vi "INFOOFMOTOR.vi"(9 "input cluster":T1, 10 "reference in":refnum<vi>, 11 "Array in":refnum<vi>) -> (3 "Mirror Info":string[](array[string]))   [LabVIEW 2013]
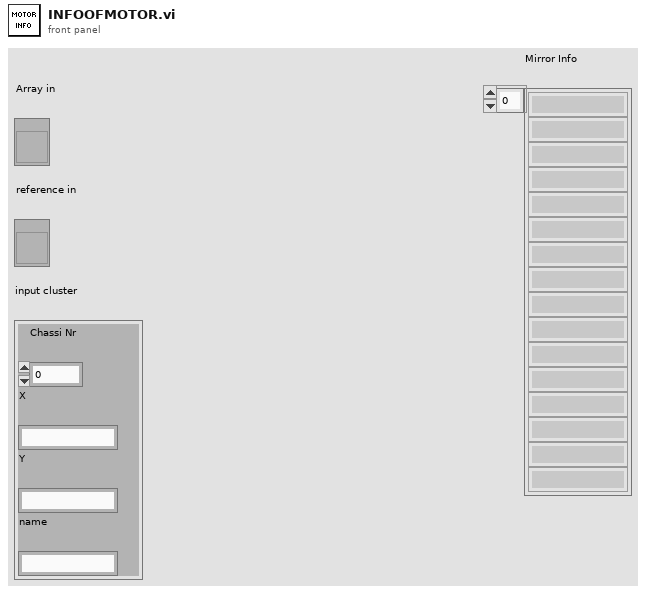
[diagram p1: front panel]
types:
  T1 = cluster{"Chassi Nr":i32, "X":string, "Y":string, "name":string}
  T2 = typedef "TRAServer.lvclass/StatusTRA_TypDef.ctl" = enum16{"NOT REFERENCED", "CONFIGURATION", "HOMING", "MOVING", "READY", "DISABLE", "JOGGING"}
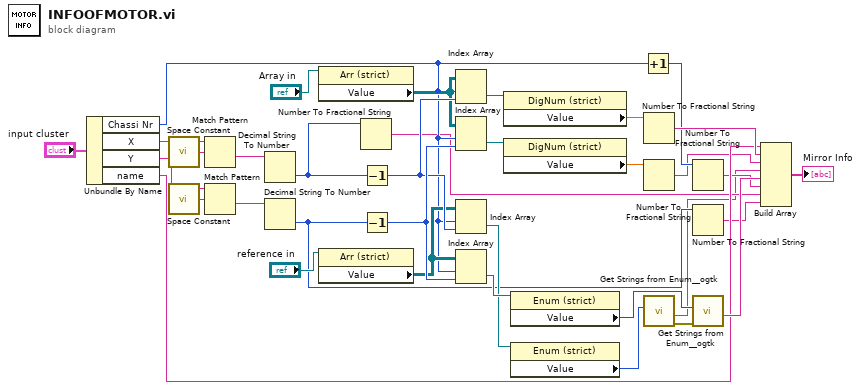
[diagram p0: block diagram]
diagram:
  n1 = Unbundle By Name("input cluster") -> ("Chassi Nr"=w9:i32, "X"=w16:string, "Y"=w20:string, "name"=w33:string)
  n2 = call <vilib>:"Space Constant.vi"() -> ("String"=w15:string)
  n3 = call <vilib>:"Space Constant.vi"() -> ("String"=w18:string)
  n4 = Match Pattern(string=w16, regular expression=w15) -> (after substring=w14:string)  [unwired: 1 in, 3 out]
  n5 = Match Pattern(string=w20, regular expression=w18) -> (after substring=w19:string)  [unwired: 1 in, 3 out]
  n6 = Decimal String To Number(string=w14) -> (number=w5:i32)  [unwired: 2 in, 1 out]
  n7 = Decimal String To Number(string=w19) -> (number=w6:i32)  [unwired: 2 in, 1 out]
  n8 = property class="Arr (strict)"(reference="Array in") -> ("Value"=w17:refnum<vi>[][])  [unwired: 1 in, 2 out]
  n9 = property class="Arr (strict)"(reference="reference in") -> ("Value"=w22:refnum<vi>[][])  [unwired: 1 in, 2 out]
  n10 = Number To Fractional String(number=w5) -> (F-format string=w3:string)  [unwired: 3 in]
  n11 = Decrement(x=w5) -> (x-1=w23:i32)
  n12 = Decrement(x=w6) -> (x-1=w24:i32)
  n13 = Index Array(array=w17, index (row)=w9, index (col)=w23) -> (element=w13:refnum<vi>)
  n14 = Index Array(array=w17, index (row)=w9, index (col)=w24) -> (element=w21:refnum<vi>)
  n15 = Index Array(array=w22, index (row)=w9, index (col)=w23) -> (element=w25:refnum<vi>)
  n16 = Index Array(array=w22, index (row)=w9, index (col)=w24) -> (element=w26:refnum<vi>)
  n17 = property class="DigNum (strict)"(reference=w13) -> ("Value"=w31:dbl)  [unwired: 1 in, 2 out]
  n18 = property class="DigNum (strict)"(reference=w21) -> ("Value"=w32:dbl)  [unwired: 1 in, 2 out]
  n19 = property class="Enum (strict)"(reference=w26) -> ("Value"=w29:T2)  [unwired: 1 in, 2 out]
  n20 = property class="Enum (strict)"(reference=w25) -> ("Value"=w27:T2)  [unwired: 1 in, 2 out]
  n21 = Increment(x=w9) -> (x+1=w8:i32)
  n22 = Number To Fractional String(number=w31) -> (F-format string=w34:string)  [unwired: 3 in]
  n23 = Number To Fractional String(number=w32) -> (F-format string=w2:string)  [unwired: 3 in]
  n24 = call <userlib>:"Get Strings from Enum__ogtk.vi"("Enum"=w27) -> ("error out"=w28:errorcluster, "String Value"=w1:string)  [unwired: 7 in, 2 out]
  n25 = Number To Fractional String(number=w8) -> (F-format string=w7:string)  [unwired: 3 in]
  n26 = Number To Fractional String(number=w6) -> (F-format string=w4:string)  [unwired: 3 in]
  n27 = call <userlib>:"Get Strings from Enum__ogtk.vi"("error in (no error)"=w28, "Enum"=w29) -> ("String Value"=w35:string)  [unwired: 6 in, 3 out]
  n28 = Build Array(w33, w34, w2, w1, w35, w7, w3, w4) -> (→"Mirror Info":string[])
